vi "_builtins_terminals_wired.vi"(11 "Terminals":refnum<vi>[](array[refnum])) -> (1 "Node Input indexes":i32[](array[numeric]), 2 "Node Output indexes":i32[](array[numeric]), 3 "Terms Wired":bool[](array[boolean]))   [LabVIEW 2019, in "Script.lvlib"]
doc: "Returns source and sink terminal indexes that are wired."
uses:
  Script.lvlib
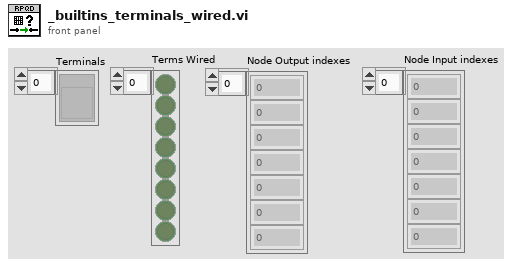
[diagram p1: front panel]
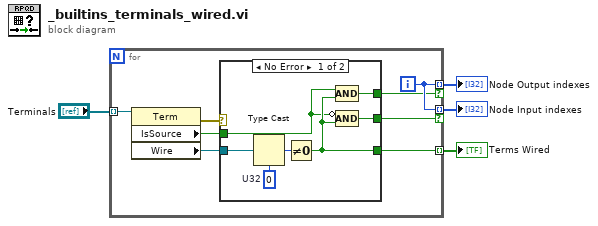
[diagram p0: block diagram]
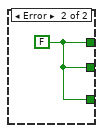
[diagram p2: hidden frame]
diagram:
  n1 = for {
    tunnel: "Terminals" -> [w11] mode=indexing
    tunnel: [w9] -> w3 mode=indexing
    tunnel: [w10] -> w2 mode=indexing if=w7
    tunnel: [w10] -> w1 mode=indexing if=w6
    i -> [w10]
    n2 = property class="Term"(reference=w11) -> (error out=w5:errorcluster, "IsSource"=w8:bool, "Wire"=w12:refnum<vi>)  [unwired: 1 in, 1 out]
    n3 = case shown="No Error" w5 {
      tunnel: w12 -> [w19 _]
      tunnel: [w16 w20] -> w9
      tunnel: w8 -> [w15 _]
      tunnel: [w14 w20] -> w7
      tunnel: [w13 w20] -> w6
      frame No Error {
        w18 = u32 0  # U32
        n4 = Type Cast(type=w18, x=w19) -> (*(type *) &x=w17:u32)
        n5 = Not Equal To 0?(x=w17) -> (x != 0?=w16:bool)
        n6 = Compound Arithmetic op=AND(w15, w16) -> (w14:bool)
        n7 = Compound Arithmetic op=AND(invert w15, w16) -> (w13:bool)
      }
      frame Error {
        w20 = FALSE
      }
    }
  }
  "Node Output indexes" <- w2
  "Node Input indexes" <- w1
  "Terms Wired" <- w3
